vi "stake master data collection MONTH WISE .vi"(0 "Refnum in":T1, 1 "STAKEHOLDER ID":string, 2 "total in date":string[](array[string]), 5 "Shift":string, 7 "Select year":string, 9 "Select Line":string, 11 "error in (no error)":errorcluster, 12 "Select month":string) -> (3 "Count out":string[](array[string]), 4 "Refnum out":T1, 6 "string min":string[](array[string]), 10 "DURATION SUM OF ARRAY":dbl, 14 "COUNT OF ARRAY":dbl, 15 "error out":errorcluster)   [LabVIEW 2017]
uses:
  <vilib>/addons/database/Connection.llb/Conn ObjectReference.ctl
  <vilib>/addons/database/NI_Database_API.lvlib
panel:
  out "output":string[][](array[string])
  out "Count out 2":string[](array[string])
  out "DURATION":string[](array[string])
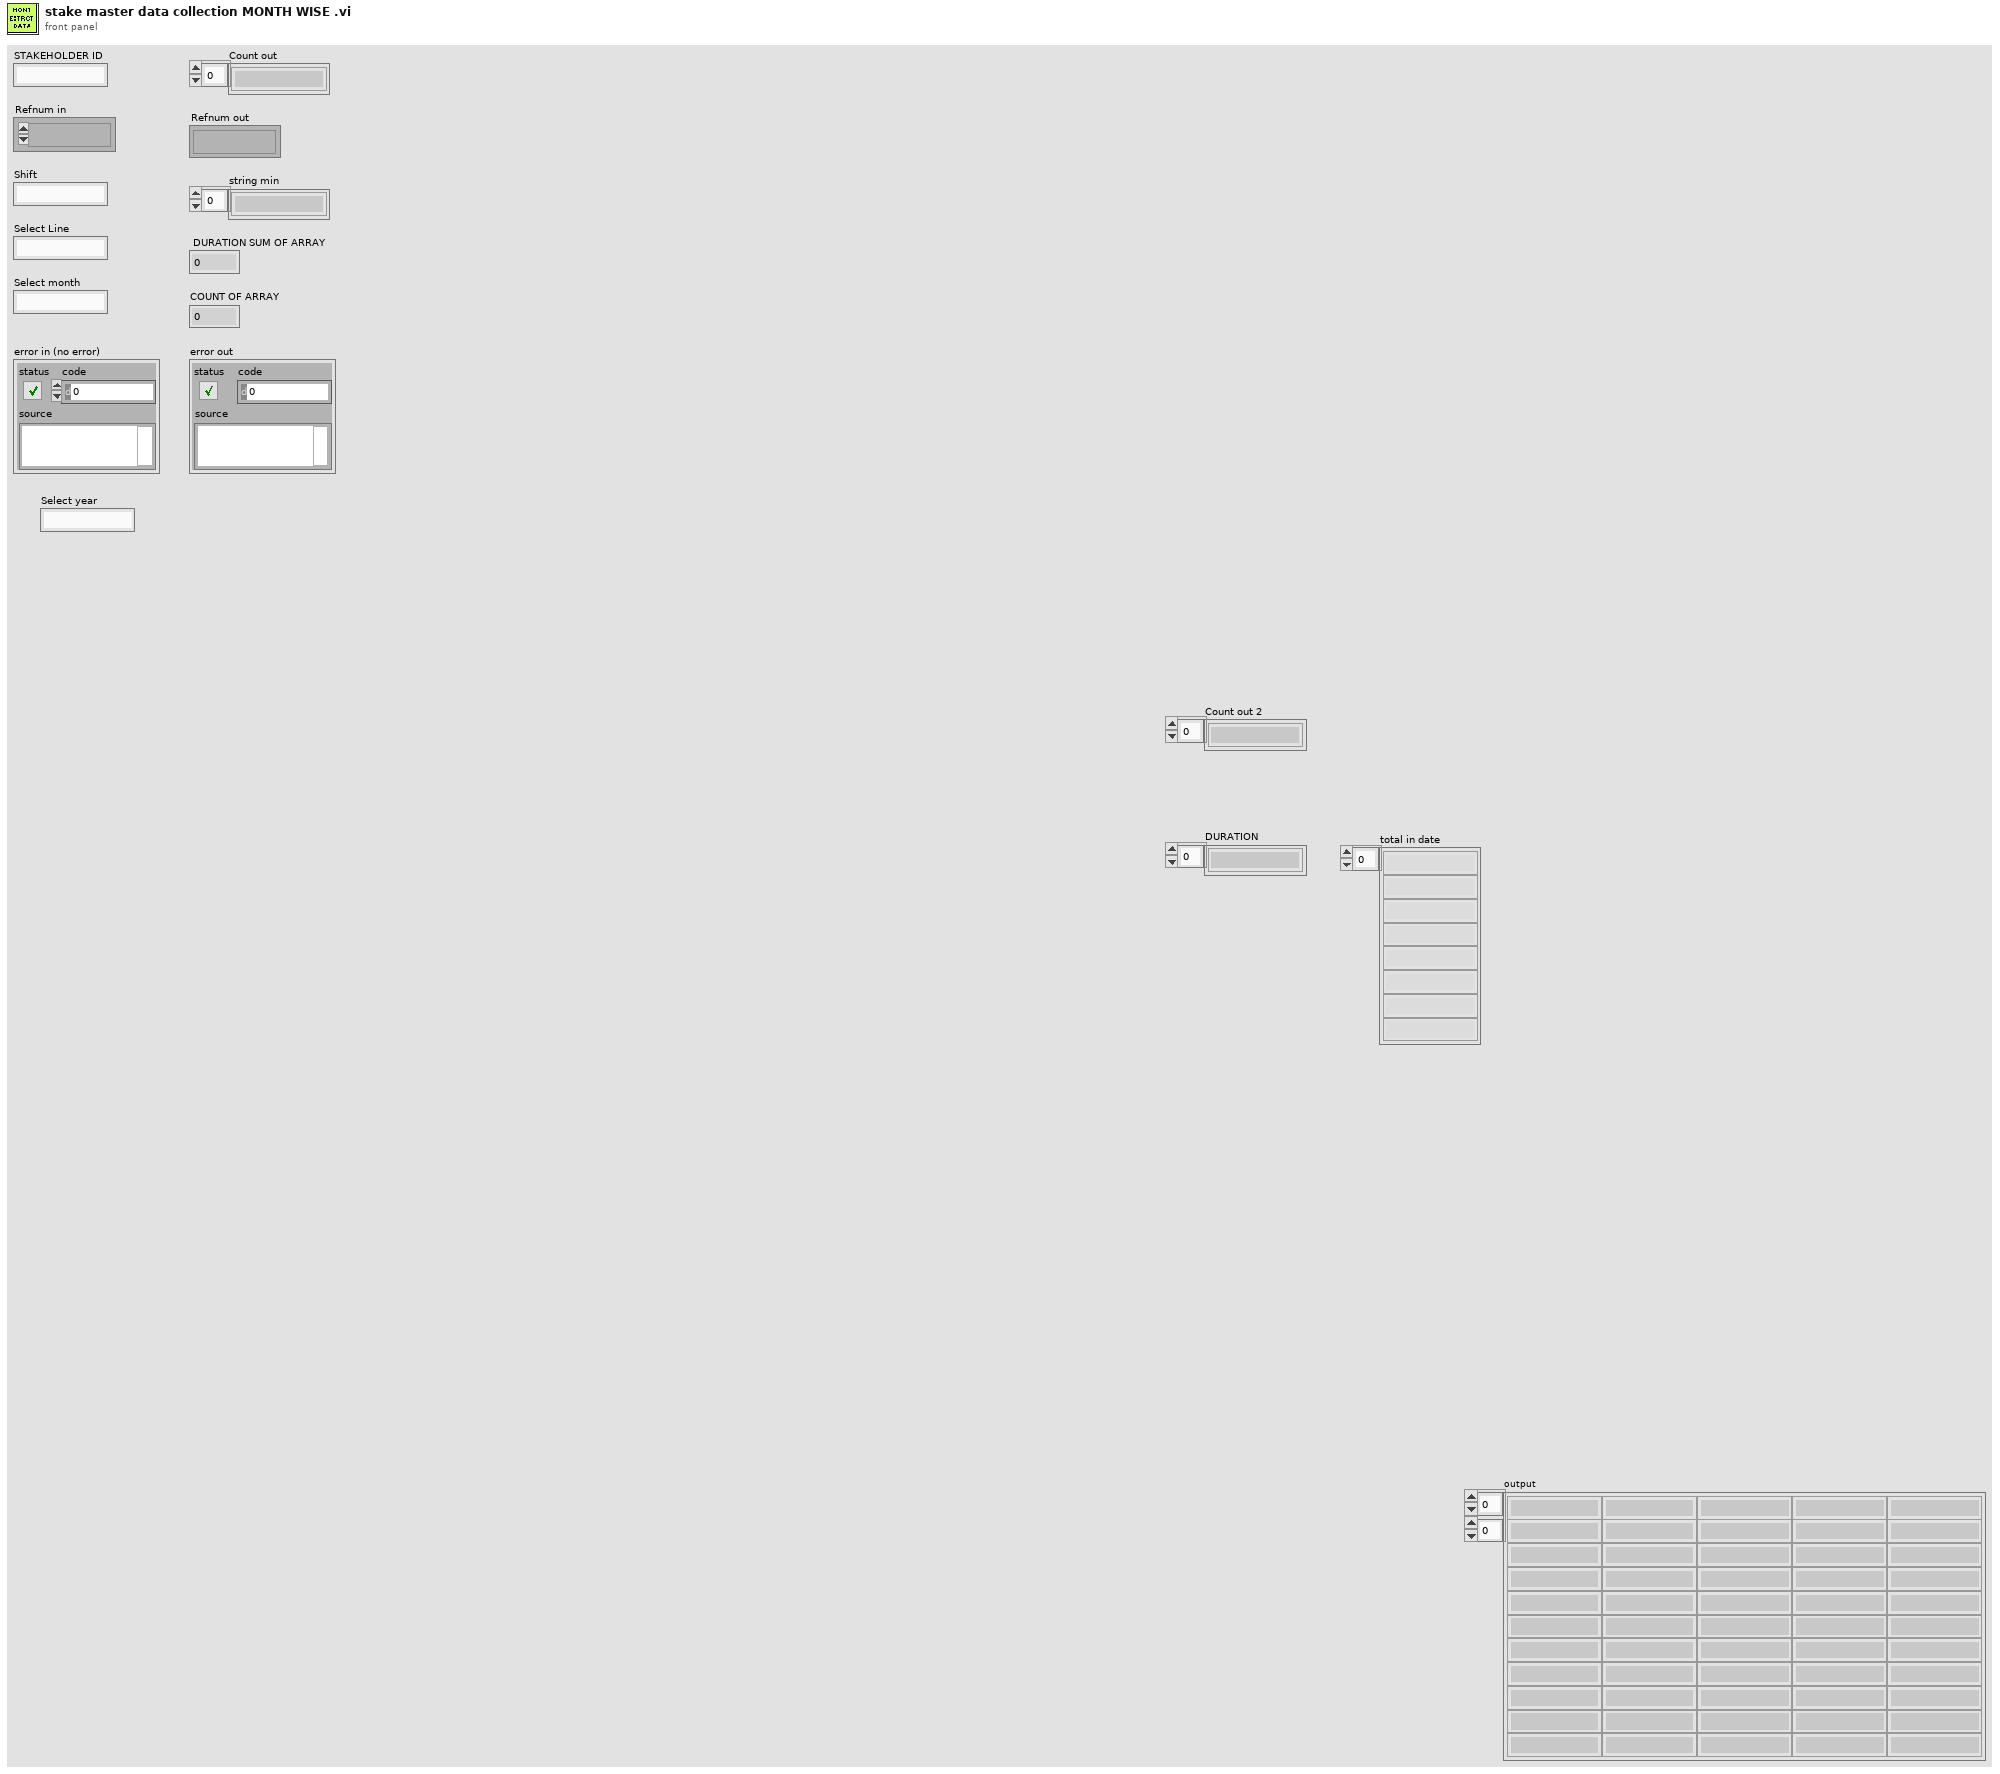
[diagram p1: front panel]
types:
  T1 = typedef "NI_Database_API.lvlib/Conn ObjectReference.ctl" = refnum<k1>
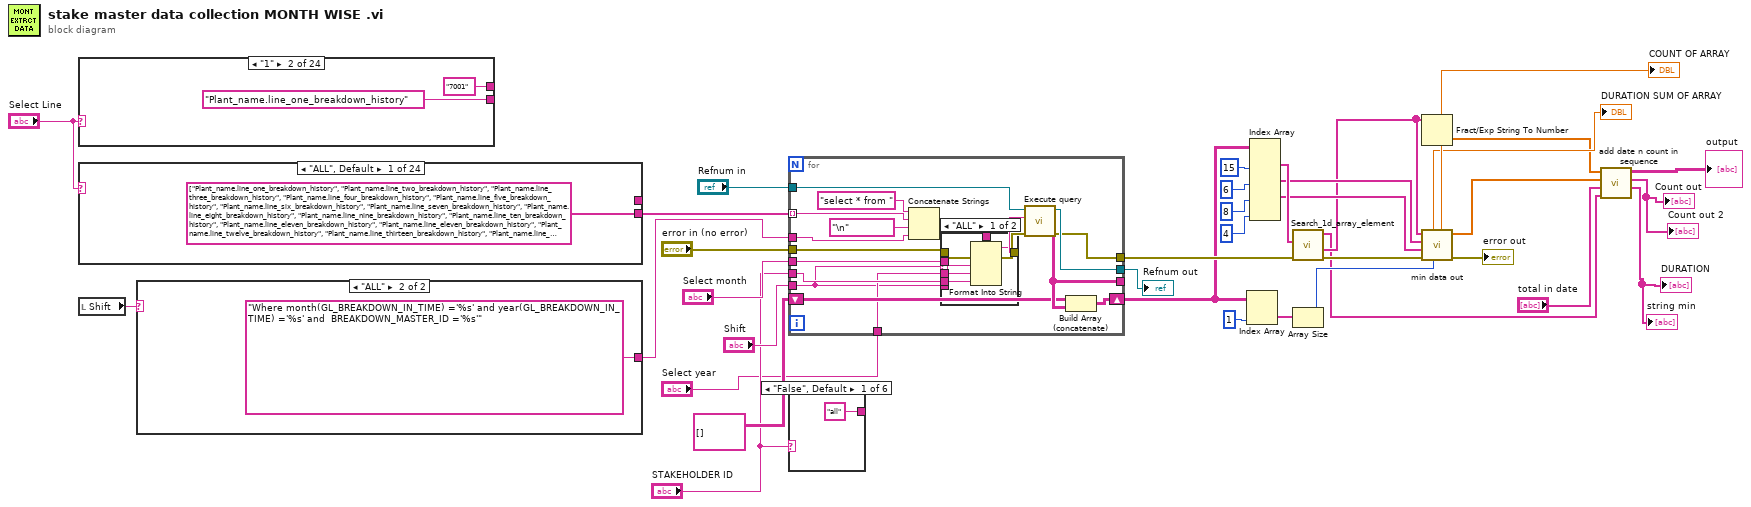
[diagram p0: block diagram]
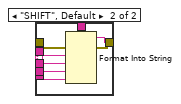
[diagram p2: hidden frame]
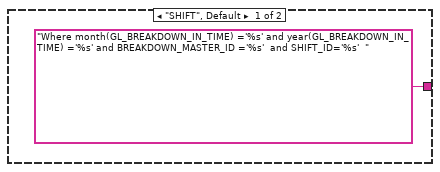
[diagram p3: hidden frame]
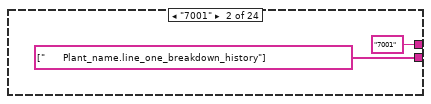
[diagram p4: hidden frame]
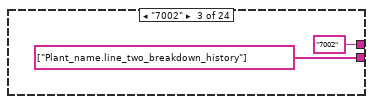
[diagram p5: hidden frame]
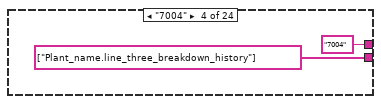
[diagram p6: hidden frame]
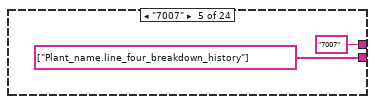
[diagram p7: hidden frame]
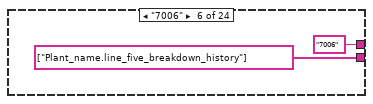
[diagram p8: hidden frame]
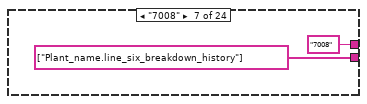
[diagram p9: hidden frame]
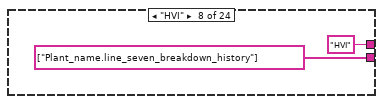
[diagram p10: hidden frame]
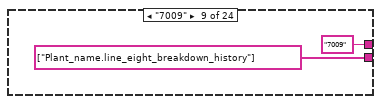
[diagram p11: hidden frame]
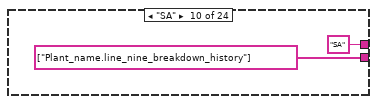
[diagram p12: hidden frame]
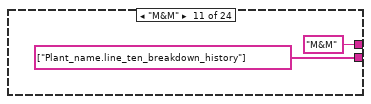
[diagram p13: hidden frame]
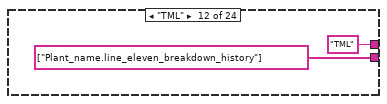
[diagram p14: hidden frame]
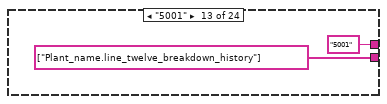
[diagram p15: hidden frame]
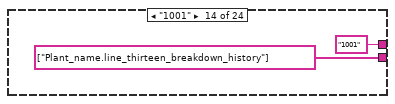
[diagram p16: hidden frame]
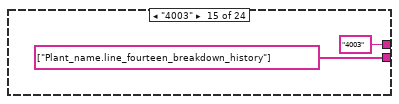
[diagram p17: hidden frame]
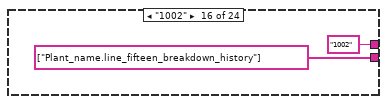
[diagram p18: hidden frame]
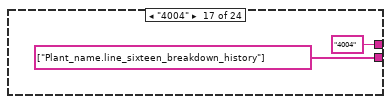
[diagram p19: hidden frame]
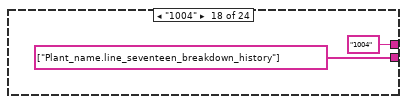
[diagram p20: hidden frame]
diagram:
  n1 = case shown="\"1\"" "Select Line" {
    tunnel: [_ "7001" "7002" "7004" "7007" "7006" "7008" "HVI" "7009" "SA" "M&M" "TML" "5001" "1001" "4003" "1002" "4004" "1004" "2001" "3001" "2004" "3002" "3003" "4001"] -> _
    tunnel: [_ "Plant_name.line_one_breakdown_history" ("table") "Plant_name.line_two_breakdown_history" ("table") "Plant_name.line_three_breakdown_history" ("table") "Plant_name.line_four_breakdown_history" ("table") "Plant_name.line_five_breakdown_history" ("table") "Plant_name.line_six_breakdown_history" ("table") "Plant_name.line_seven_breakdown_history" ("table") "Plant_name.line_eight_breakdown_history" ("table") "Plant_name.line_nine_breakdown_history" ("table") "Plant_name.line_ten_breakdown_history" ("table") "Plant_name.line_eleven_breakdown_history" ("table") "Plant_name.line_twelve_breakdown_history" ("table") "Plant_name.line_thirteen_breakdown_history" ("table") "Plant_name.line_fourteen_breakdown_history" ("table") "Plant_name.line_fifteen_breakdown_history" ("table") "Plant_name.line_sixteen_breakdown_history" ("table") "Plant_name.line_seventeen_breakdown_history" ("table") "Plant_name.line_eighteen_breakdown_history" ("table") "Plant_name.line_nineteen_breakdown_history" ("table") "Plant_name.line_twenty_breakdown_history" ("table") "Plant_name.line_twenty_one_breakdown_history" ("table") "Plant_name.line_twenty_two_breakdown_history" ("table") "Plant_name.line_twenty_three_breakdown_history" ("table")] -> _
    frame "0", Default {
    }
    frame "1" {
    }
    frame "2" {
    }
    frame "3" {
    }
    frame "4" {
    }
    frame "5" {
    }
    frame "6" {
    }
    frame "7" {
    }
    frame "8" {
    }
    frame "9" {
    }
    frame "10" {
    }
    frame "11" {
    }
    frame "12" {
    }
    frame "13" {
    }
    frame "14" {
    }
    frame "15" {
    }
    frame "16" {
    }
    frame "17" {
    }
    frame "18" {
    }
    frame "19" {
    }
    frame "20" {
    }
    frame "21" {
    }
    frame "22" {
    }
    frame "23" {
    }
  }
  n2 = case shown="\"ALL\", Default" "Select Line" {
    tunnel: [_ "7001" "7002" "7004" "7007" "7006" "7008" "HVI" "7009" "SA" "M&M" "TML" "5001" "1001" "4003" "1002" "4004" "1004" "2001" "3001" "2004" "3002" "3003" "4001"] -> _
    tunnel: [string[] ["Plant_name.line_one_breakdown_history", "Plant_name.line_two_breakdown_history", "Plant_name.line_three_breakdown_history", "Plant_name.line_four_breakdown_history", "Plant_name.line_five_breakdown_history", "Plant_name.line_six_breakdown_history", "Plant_name.line_seven_breakdown_history", "Plant_name.line_eight_breakdown_history", "Plant_name.line_nine_breakdown_history", "Plant_name.line_ten_breakdown_history", "Plant_name.line_eleven_breakdown_history", "Plant_name.line_eleven_breakdown_history", "Plant_name.line_twelve_breakdown_history", "Plant_name.line_thirteen_breakdown_history", "Plant_name.line_fourteen_breakdown_history", "Plant_name.line_fifteen_breakdown_history", "Plant_name.line_sixteen_breakdown_history", "Plant_name.line_seventeen_breakdown_history", "Plant_name.line_eighteen_breakdown_history", "Plant_name.line_nineteen_breakdown_history", "Plant_name.line_twenty_breakdown_history", "Plant_name.line_twenty_one_breakdown_history", "Plant_name.line_twenty_two_breakdown_history", "Plant_name.line_twenty_three_breakdown_history"] string[] ["      Plant_name.line_one_breakdown_history"] string[] ["Plant_name.line_two_breakdown_history"] string[] ["Plant_name.line_three_breakdown_history"] string[] ["Plant_name.line_four_breakdown_history"] string[] ["Plant_name.line_five_breakdown_history"] string[] ["Plant_name.line_six_breakdown_history"] string[] ["Plant_name.line_seven_breakdown_history"] string[] ["Plant_name.line_eight_breakdown_history"] string[] ["Plant_name.line_nine_breakdown_history"] string[] ["Plant_name.line_ten_breakdown_history"] string[] ["Plant_name.line_eleven_breakdown_history"] string[] ["Plant_name.line_twelve_breakdown_history"] string[] ["Plant_name.line_thirteen_breakdown_history"] string[] ["Plant_name.line_fourteen_breakdown_history"] string[] ["Plant_name.line_fifteen_breakdown_history"] string[] ["Plant_name.line_sixteen_breakdown_history"] string[] ["Plant_name.line_seventeen_breakdown_history"] string[] ["Plant_name.line_eighteen_breakdown_history"] string[] ["Plant_name.line_nineteen_breakdown_history"] string[] ["Plant_name.line_twenty_breakdown_history"] string[] ["Plant_name.line_twenty_one_breakdown_history"] string[] ["Plant_name.line_twenty_two_breakdown_history"] string[] ["Plant_name.line_twenty_three_breakdown_history"]] -> w13
    frame "ALL", Default {
    }
    frame "7001" {
    }
    frame "7002" {
    }
    frame "7004" {
    }
    frame "7007" {
    }
    frame "7006" {
    }
    frame "7008" {
    }
    frame "HVI" {
    }
    frame "7009" {
    }
    frame "SA" {
    }
    frame "M&M" {
    }
    frame "TML" {
    }
    frame "5001" {
    }
    frame "1001" {
    }
    frame "4003" {
    }
    frame "1002" {
    }
    frame "4004" {
    }
    frame "1004" {
    }
    frame "2001" {
    }
    frame "3001" {
    }
    frame "2004" {
    }
    frame "3002" {
    }
    frame "3003" {
    }
    frame "4001" {
    }
  }
  n3 = local read "Shift"() -> (w14:string)
  n4 = case shown="\"ALL\"" w14 {
    tunnel: ["Where month(GL_BREAKDOWN_IN_TIME) ='%s' and year(GL_BREAKDOWN_IN_TIME) ='%s' and BREAKDOWN_MASTER_ID ='%s'  and SHIFT_ID='%s'  " ("condition") "Where month(GL_BREAKDOWN_IN_TIME) ='%s' and year(GL_BREAKDOWN_IN_TIME) ='%s' and  BREAKDOWN_MASTER_ID ='%s'" ("condition")] -> w35
    frame "SHIFT", Default {
    }
    frame "ALL" {
    }
  }
  n5 = for {
    tunnel: "Select month" -> [w149]
    tunnel: w35 -> [w148]
    tunnel: [w137] -> _
    tunnel: "Shift" -> [w132]
    tunnel: w13 -> [w138] mode=indexing
    tunnel: "STAKEHOLDER ID" -> [w134]
    tunnel: "Refnum in" -> [w139]
    tunnel: [w147] -> w34
    tunnel: "error in (no error)" -> [w140]
    tunnel: [w146] -> w33
    shift-right: [w136] -> w11
    shift-left: string[][] [] -> [w135]
    tunnel: "Select year" -> [w133]
    n6 = Concatenate Strings("select * from " ("string"), w138, "\n" ("string"), w148) -> (w142:string)
    n7 = case shown="\"ALL\"" w132 {
      tunnel: w149 -> [w156 w164]
      tunnel: [w155 w163] -> w144
      tunnel: [w154 w162] -> w143
      tunnel: w142 -> [w153 w161]
      tunnel: w132 -> [_ w160]
      tunnel: w140 -> [w152 w159]
      tunnel: w134 -> [w151 w158]
      tunnel: w133 -> [w150 w157]
      frame "ALL" {
        n8 = Format Into String(format string=w153, error in=w152, w156, w150, w151) -> (resulting string=w155:string, error out=w154:errorcluster)  [unwired: 1 in]
      }
      frame "SHIFT", Default {
        n9 = Format Into String(format string=w161, error in=w159, w164, w157, w158, w160) -> (resulting string=w163:string, error out=w162:errorcluster)  [unwired: 1 in]
      }
    }
    n10 = call "Execute query.vi"("error in (no error)"=w143, "String"=w144, "connection reference"=w139) -> ("error out"=w146:errorcluster, "Table"=w137:string[][], "connection reference 2"=w147:T1)  [unwired: 5 in, 1 out]
    n11 = Build Array (concatenate)(w135, w137) -> (w136:string[][])
  }
  "Refnum out" <- w34
  n12 = case shown="\"False\", Default" "STAKEHOLDER ID" {
    tunnel: ["all" "1" "2" "3" "4" "5"] -> _
    frame "False", Default {
    }
    frame "Logistics" {
    }
    frame "Maintenance" {
    }
    frame "Quality" {
    }
    frame "Production" {
    }
    frame "Gap Leader" {
    }
  }
  n13 = Index Array(array=w11, index (col)=1 ("disabled index (col)")) -> (element=w22:string[])  [unwired: 1 in]
  n14 = Index Array(array=w11, index (col) #1=15 ("index (row)"), index (col) #2=6 ("index (col)"), index (col) #3=8 ("index (col)"), index (col) #4=4 ("index (col)")) -> (element #1=w28:string[], element #2=w23:string[], element #3=w24:string[])  [unwired: 4 in, 1 out]
  n15 = call "Search_1d_array_element.vi"("error in (no error)"=w33, "BD Date"=w28) -> ("error out"=w27:errorcluster, "Count out"=w7:string[], "Elements Found out"=w4:string[])  [unwired: 5 in]
  n16 = Array Size(array=w22) -> (size(s)=w25:i32)
  n17 = Fract/Exp String To Number(string=w7) -> (number=w6:dbl[])  [unwired: 3 in, 1 out]
  n18 = call "min data out.vi"("Numeric"=w25, "error in (no error)"=w27, "out time"=w24, "in time"=w23, "Count in"=w7) -> ("error out"=→"error out":errorcluster, "duration"=w5:dbl[], "COUNT OF ARRAY"=→"COUNT OF ARRAY":dbl, "DURATION SUM OF ARRAY"=→"DURATION SUM OF ARRAY":dbl)  [unwired: 2 in, 1 out]
  n19 = call "add date n count in sequence.vi"("find date"=w4, "total date"="total in date", "duration"=w5, "count"=w6) -> ("DURATION"=→"string min" →"DURATION":string[], "COUNT"=→"Count out" →"Count out 2":string[], "appended array"=→"output":string[][])  [unwired: 5 in]
